vi "Start Calculation.vi"(8 "error in (no error)":errorcluster, 11 "CPU FFT Calculator in":refnum<class "CPU FFT Calculator.lvclass">) -> (0 "error out":errorcluster, 3 "CPU FFT Calculator out":refnum<class "CPU FFT Calculator.lvclass">)   [LabVIEW 2020, in "CPU FFT Calculator.lvlib" / "CPU FFT Calculator.lvclass"]
uses:
  CPU FFT Calculator.lvclass
  C:/Users/natan/Documents/G2CPU-Performance-Demo/Calculation Worker/Calculation Worker/Calculation Worker.lvclass
  C:/Program Files/National Instruments/LabVIEW 2026/vi.lib/ActorFramework/Actor/Actor.lvclass
  <vilib>/ActorFramework/Actor/Actor.lvclass/Actor.ctl
  <vilib>/ActorFramework/Message Enqueuer/Message Enqueuer.lvclass/Message Enqueuer.ctl
  Application Manager/Application Manager Messages/Set UI CPU Done Msg/Set UI CPU Done Msg.lvclass/Set UI CPU Done Msg.ctl
  <vilib>/ActorFramework/Message Enqueuer/Init from Existing Queue.vi
  <vilib>/ActorFramework/Message Enqueuer/Enqueue.vi
  CPU FFT Calculator Messages/Do Calculation Msg/Do Calculation Msg.lvclass
  C:/Program Files/National Instruments/LabVIEW 2026/vi.lib/ActorFramework/Message/Message.lvclass
  Application Manager/Application Manager Messages/Set UI CPU Done Msg/Set UI CPU Done Msg.lvclass
  <vilib>/ActorFramework/Message Priority Queue/Priority Enqueue.vi
  <vilib>/ActorFramework/Message Enqueuer/Message Enqueuer.lvclass
  <vilib>/ActorFramework/Actor/Actor.lvclass
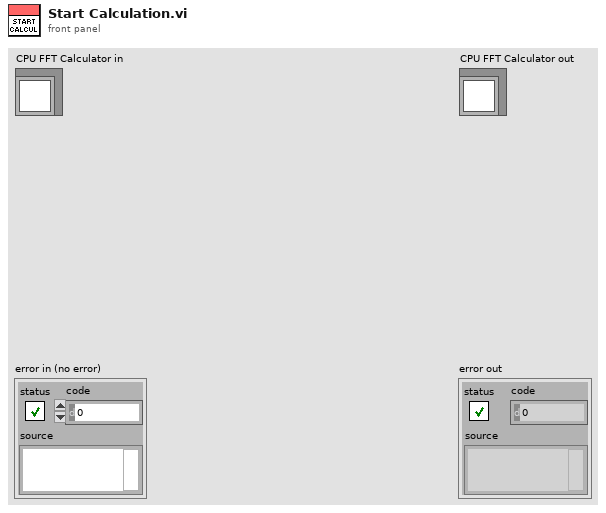
[diagram p1: front panel]
types:
  T1 = typedef "Data Source.lvlib/Data Source.lvclass/Data Source Buffer.ctl" = refnum<data-value>
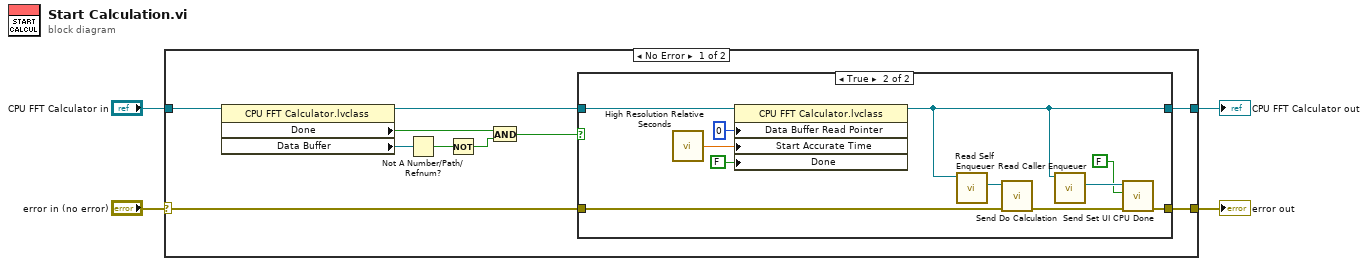
[diagram p0: block diagram]
diagram:
  n1 = case shown="No Error" "error in (no error)" {
    selector: "error in (no error)" -> [w13 w29]
    tunnel: [w11 w29] -> w3
    tunnel: [w12 w28] -> w1
    tunnel: "CPU FFT Calculator in" -> [w14 w28]
    frame No Error {
      n2 = property class="CPU FFT Calculator.lvclass"(reference=w14) -> (reference out=w10:refnum<class "CPU FFT Calculator.lvclass">, "Done"=w6:bool, "Data Buffer"=w9:T1)  [unwired: 1 in, 1 out]
      n3 = Not A Number/Path/Refnum?(number/path/refnum=w9) -> (NaN/Path/Refnum?=w8:bool)
      n4 = Not(x=w8) -> (.not. x?=w7:bool)
      n5 = And(x=w6, y=w7) -> (x .and. y?=w5:bool)
      n6 = case shown="True" w5 {
        tunnel: w13 -> [w15 w26]
        tunnel: [w16 w22] -> w12
        tunnel: [w15 w19] -> w11
        tunnel: w10 -> [w16 w17]
        frame False {
        }
        frame True {
          n7 = call <vilib>:"High Resolution Relative Seconds.vi"() -> ("relative seconds"=w24:dbl)
          n8 = property class="CPU FFT Calculator.lvclass"(reference=w17, "Data Buffer Read Pointer"=u64 0, "Start Accurate Time"=w24, "Done"=FALSE) -> (reference out=w22:refnum<class "CPU FFT Calculator.lvclass">)  [unwired: 1 in, 1 out]
          n9 = call <vilib>:"Read Self Enqueuer.vi"("Actor"=w22) -> ("Self Enqueuer"=w25:refnum<class "Message Enqueuer.lvclass">)  [unwired: 10 in]
          n10 = call "Send Do Calculation.vi"("error in (no error)"=w26, "Message Enqueuer"=w25) -> ("error out"=w20:errorcluster)  [unwired: 8 in, 1 out]
          n11 = call <vilib>:"Read Caller Enqueuer.vi"("Actor"=w22) -> ("Caller Enqueuer"=w21:refnum<class "Message Enqueuer.lvclass">)  [unwired: 10 in]
          n12 = call "Send Set UI CPU Done.vi"("error in (no error)"=w20, "CPU Done"=FALSE, "Message Enqueuer"=w21) -> ("error out"=w19:errorcluster)  [unwired: 7 in, 1 out]
        }
      }
    }
    frame Error {
    }
  }
  "error out" <- w3
  "CPU FFT Calculator out" <- w1
